vi "Flatten Parameters.vi"(0 "Executioner in":refnum<class "Executioner.lvclass">, 1 "Linked List Ref":refnum<data-value>, 5 "Active Unique ID":string, 7 "Indent":i32, 9 "Path":path, 11 "error in (no error)":errorcluster, 12 "Persistence in":refnum<class "IPersist.lvclass">) -> (3 "Linked List Ref out":refnum<data-value>, 4 "Flattened Test Executive":string[](array[string]), 8 "Active Unique ID out":string, 14 "Persistence out":refnum<class "IPersist.lvclass">, 15 "error out":errorcluster)   [LabVIEW 2017, in "Test Executive.lvlib" / "Executioner.lvclass"]
uses:
  <vilib>/gpm_packages/@cs/test-executive/Source/Test Executive/Executioner/Executioner.lvclass
  <vilib>/gpm_packages/@cs/linked-list/Source/Linked List/ILinkedList/ILinked List.lvclass
  <vilib>/gpm_packages/@cs/persistence/source/IPersist/IPersist.lvclass
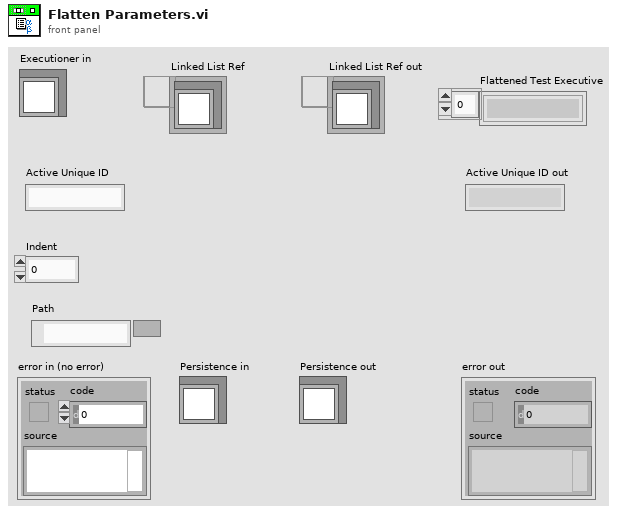
[diagram p1: front panel]
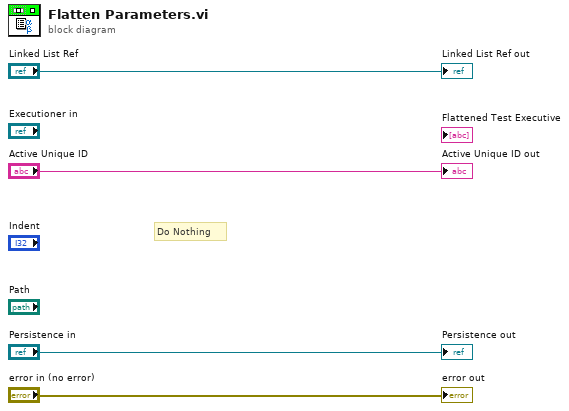
[diagram p0: block diagram]
diagram:
  # "Do Nothing"
  "error out" <- "error in (no error)"
  "Linked List Ref out" <- "Linked List Ref"
  "Active Unique ID out" <- "Active Unique ID"
  "Persistence out" <- "Persistence in"
